vi "图像采样2.vi"() -> ()   [LabVIEW 2018]
uses:
  <vilib>/vision/NI_Vision_Development_Module.lvlib
panel:
  out "Image 6":T1(plugin-control)
  out "Image 5":T1(plugin-control)
  out "Image 4":T1(plugin-control)
  out "Image 3":T1(plugin-control)
  out "error out":errorcluster
  out "Image 2":T1(plugin-control)
  out "Image":T1(plugin-control)
  in  "路径":path
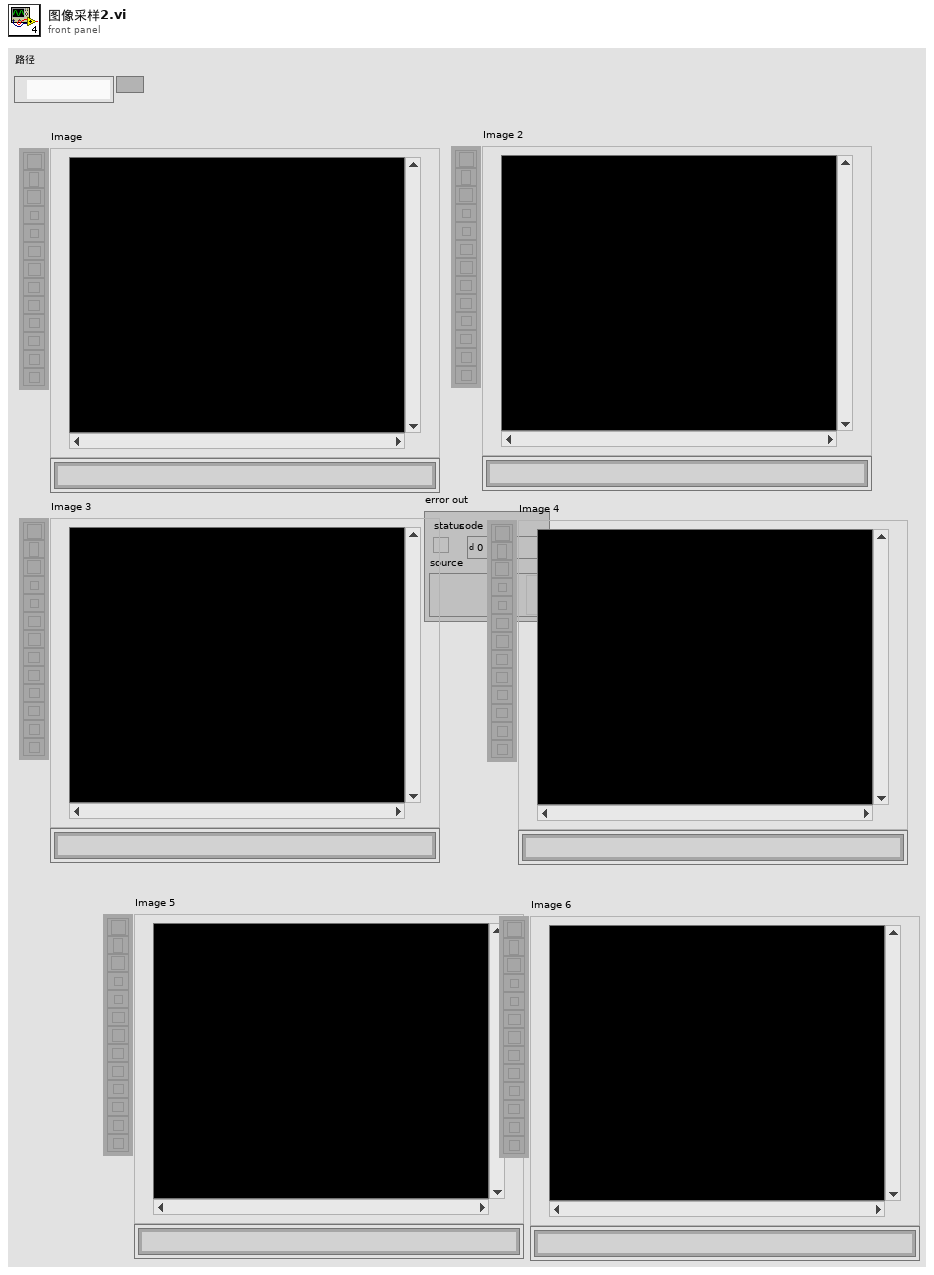
[diagram p1: front panel]
types:
  T1 = typedef "IMAQ Image.ctl" = refnum<image>
  T2 = cluster{"Interpolation Type":enum32{"Zero Order", "Bilinear", "Quadratic", "Cubic", "Bilinear Fixed"}, "Destination Width":u32, "Destination Height":u32, "Fill Value":sgl}
  T3 = typedef "ROI Descriptor" = cluster{"Global Rectangle":i32[], "Contours":cluster{"ID":enum32{"External", "Internal"}, "Type":u32, "Coordinates":i32[]}[]}
  T4 = typedef "Image Type" = u32
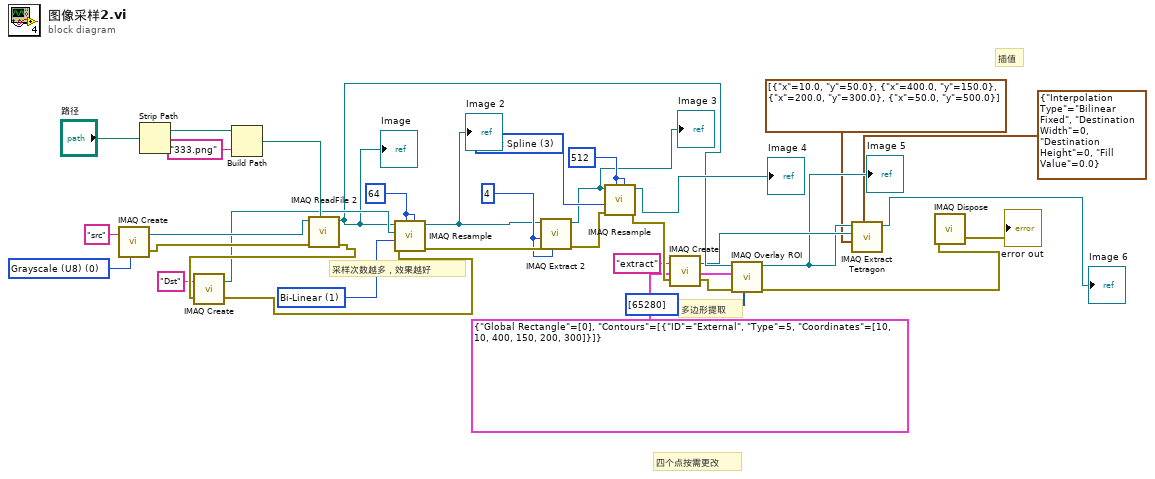
[diagram p0: block diagram]
diagram:
  w17 = 512 ("Y Resolution")
  w18 = u32 3 items=["Zero Order", "Bi-Linear", "Quadratic", "Cubic Spline"] ("Interpolation Type")
  w19 = 4 ("X Step Size")
  w26 = u32 1 items=["Zero Order", "Bi-Linear", "Quadratic", "Cubic Spline"] ("Interpolation Type")
  w27 = 64 ("Y Resolution")
  w29 = T4 0 items=["Grayscale (U8)", "Grayscale (I16)", "Grayscale (SGL)", "Complex (CSG)", "RGB (U32)", "HSL (U32)", "RGB (U64)", "Grayscale (U16)"] ("Image Type")
  # "四个点按需更改"
  # "插值"
  # "多边形提取"
  # "采样次数越多，效果越好"
  n1 = call "IMAQ Create"("Image Name"="src", "Image Type"=w29) -> ("New Image"=w32:T1, "error out"=w31:errorcluster)  [unwired: 3 in]
  n2 = Strip Path(path="路径") -> (stripped path=w34:path)  [unwired: 1 out]
  n3 = Build Path(base path=w34, name or relative path="333.png" ("名称或相对路径")) -> (appended path=w28:path)
  n4 = call "IMAQ ReadFile 2"("File Path"=w28, "error in (no error)"=w31, "Image"=w32) -> ("error out"=w25:errorcluster, "Image Out"=w10:T1)  [unwired: 4 in, 3 out]
  "Image" <- w10
  n5 = call "IMAQ Create"("Image Name"="Dst", "error in (no error)"=w25) -> ("New Image"=w23:T1, "error out"=w24:errorcluster)  [unwired: 3 in]
  n6 = call "IMAQ Resample"("X Resolution"=w27, "Y Resolution"=w27, "error in (no error)"=w24, "Interpolation Type"=w26, "Image Dst"=w23, "Image Src"=w10) -> ("error out"=w21:errorcluster, "Image Dst Out"=w16:T1)  [unwired: 4 in]
  "Image 2" <- w16
  n7 = call "IMAQ Extract 2"("Y Step Size"=w19, "error in (no error)"=w21, "X Step Size"=w19, "Image Src"=w16) -> ("error out"=w13:errorcluster, "Image Dst Out"=w15:T1)  [unwired: 6 in]
  "Image 3" <- w15
  n8 = call "IMAQ Resample"("X Resolution"=w17, "Y Resolution"=w17, "error in (no error)"=w13, "Interpolation Type"=w18, "Image Src"=w15) -> ("error out"=w12:errorcluster, "Image Dst Out"=→"Image 4":T1)  [unwired: 5 in]
  n9 = call "IMAQ Create"("Image Name"="extract", "error in (no error)"=w12) -> ("New Image"=w5:T1, "error out"=w8:errorcluster)  [unwired: 3 in]
  n10 = call "IMAQ Overlay ROI"("Colors (Green)"=u32[] [65280], "error in (no error)"=w8, "ROI Descriptor"=T3 {"Global Rectangle"=[0], "Contours"=[{"ID"=enum."External", "Type"=5, "Coordinates"=[10, 10, 400, 150, 200, 300]}]}, "Image"=w10) -> ("error out"=w6:errorcluster, "Image Out"=w4:T1)  [unwired: 6 in]
  "Image 5" <- w4
  n11 = call-poly "IMAQ Extract Tetragon"("Options"=T2 {"Interpolation Type"=enum."Bilinear Fixed", "Destination Width"=0, "Destination Height"=0, "Fill Value"=0.0}, "Tetragon"=cluster{"x":sgl, "y":sgl}[] [{"x"=10.0, "y"=50.0}, {"x"=400.0, "y"=150.0}, {"x"=200.0, "y"=300.0}, {"x"=50.0, "y"=500.0}], "Image Dst"=w5, "Image Src"=w4) -> ("Image Dst Out"=→"Image 6":T1)  [unwired: 6 in, 1 out]
  n12 = call "IMAQ Dispose"("error in (no error)"=w6) -> ("error out"=→"error out":errorcluster)  [unwired: 5 in]
